vi "AVI Path Gen.vi"(8 "error in (no error)":errorcluster, 9 "Frames Per Second":u32=30, 11 "Output file path":path=path "C:/Users/Teo/Desktop/UCL Datasets/160915_13_48_57 FunctAcq-6 patches") -> (0 "error out":errorcluster, 2 "Codec used":string, 3 "AVI Refnum":T1)   [LabVIEW 2017]
uses:
  <vilib>/vision/Avi.llb/IMAQ AVI2 Refnum.ctl
  Globals/gl_8-bit montage window ctrl refs.vi
panel:
  out "name":string
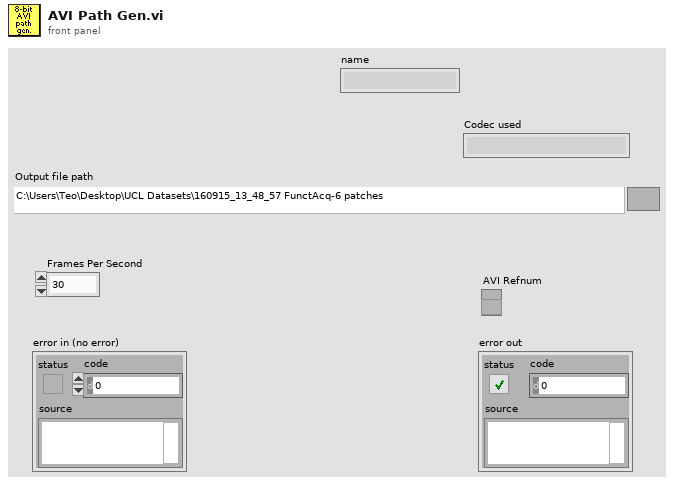
[diagram p1: front panel]
types:
  T1 = typedef "IMAQ AVI2 Refnum.ctl" = refnum<k20>
  T2 = typedef "8-bit video export window ctrl refs.ctl" = cluster{"This VI":refnum<vi>, "Add speed data":refnum<vi>, "Add camera videos":refnum<vi>, "Stop button":refnum<vi>, "Camera Video Adjustments":refnum<vi>, "Microscope Image Adjustments":refnum<vi>, "Execute":refnum<vi>, "Codec":refnum<vi>, "Channel to load":refnum<vi>, "Speed graph behaviour":refnum<vi>, "Include speed graph":refnum<vi>, "Number of rows to generate":refnum<vi>, "Path":refnum<vi>}
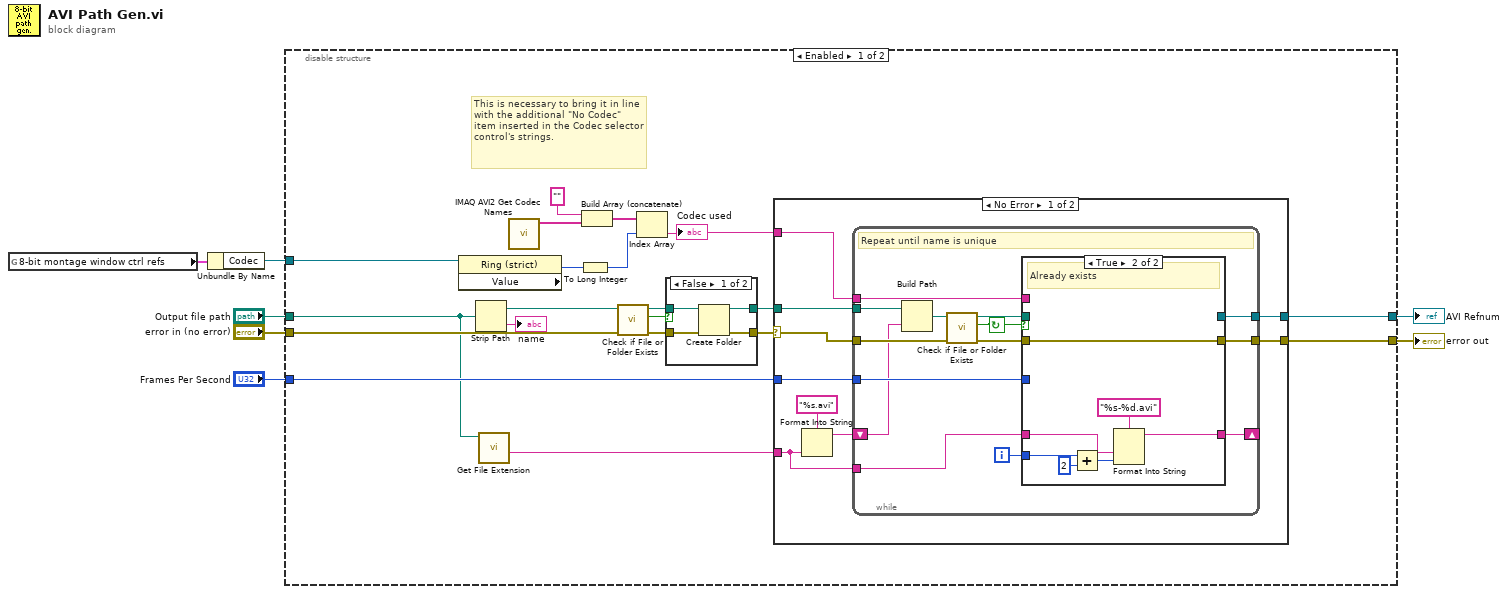
[diagram p0: block diagram]
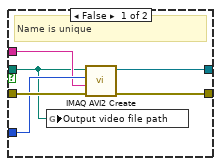
[diagram p2: hidden frame]
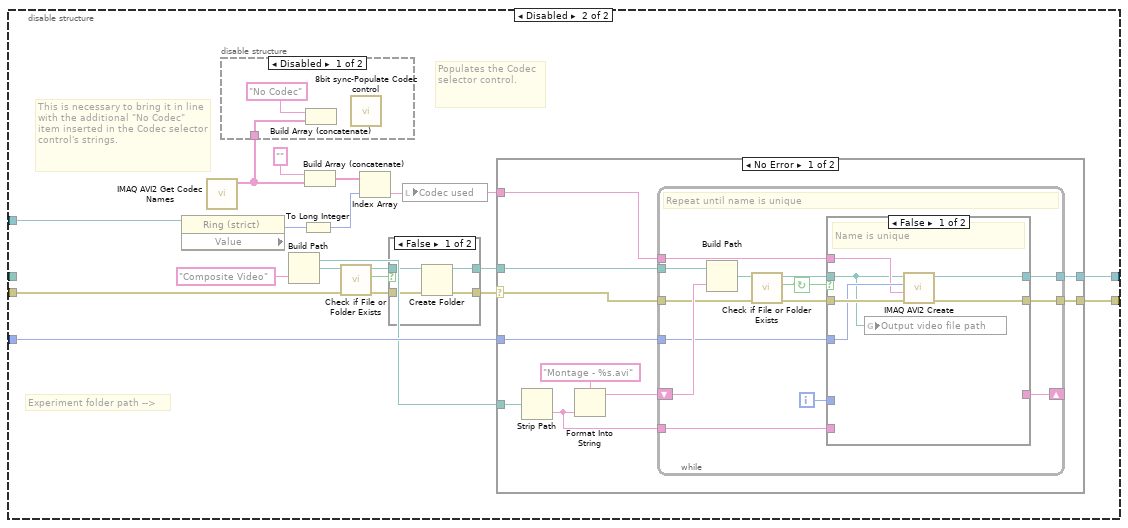
[diagram p5: hidden frame]
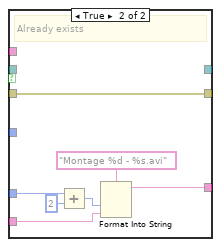
[diagram p7: hidden frame]
diagram:
  n1 = global read "gl_8-bit montage window ctrl refs.vi" "8-bit montage window ctrl refs"() -> (w3:T2)
  n2 = Unbundle By Name(w3) -> ("Codec"=w2:refnum<vi>)
  n3 = disable-structure shown="Enabled" {
    disable-tunnel: "Frames Per Second" -> [w22 w83]
    disable-tunnel: [w21 w82] -> w6
    disable-tunnel: "error in (no error)" -> [w19 w80]
    disable-tunnel: [w18 w79] -> w4
    disable-tunnel: w2 -> [w13 w75]
    disable-tunnel: "Output file path" -> [w9 _]
    frame Enabled {
      # "This is necessary to bring it in line with the additional \"No Codec\" item inserted in the Codec selector control's strings."
      n4 = property class="Ring (strict)"(reference=w13) -> ("Value"=w12:u16)  [unwired: 1 in, 2 out]
      n5 = Strip Path(path=w9) -> (stripped path=w27:path, name=→"name":string)
      n6 = call <vilib>:"Get File Extension.vi"("file"=w9) -> ("filename without extension"=w8:string)  [unwired: 6 in, 4 out]
      n7 = call "IMAQ AVI2 Get Codec Names"() -> ("Codec Names"=w15:string[])  [unwired: 10 in, 1 out]
      n8 = To Long Integer(number=w12) -> (32bit integer=w11:i32)
      n9 = Build Array (concatenate)("" ("Codec Name"), w15) -> (w14:string[])
      n10 = call <vilib>:"Check if File or Folder Exists.vi"("error in (no error)"=w19, "path"=w27) -> ("error out"=w26:errorcluster, "file or folder exists?"=w24:bool, "dup path"=w25:path)  [unwired: 7 in]
      n11 = Index Array(array=w14, index=w11) -> (element=w16:string)
      "Codec used" <- w16
      n12 = case shown="False" w24 {
        tunnel: w25 -> [w67 w70]
        tunnel: [w68 w70] -> w23
        tunnel: w26 -> [w66 w69]
        tunnel: [w65 w69] -> w20
        frame False {
          n13 = Create Folder(path (use dialog)=w67, error in=w66) -> (created path=w68:path, error out=w65:errorcluster)  [unwired: 1 in, 1 out]
        }
        frame True {
        }
      }
      n14 = case shown="No Error" w20 {
        selector: w20 -> [w30 w64]
        tunnel: w23 -> [w36 _]
        tunnel: w22 -> [w33 _]
        tunnel: [w32 _] -> w21
        tunnel: [w31 w64] -> w18
        tunnel: w16 -> [w29 _]
        tunnel: w8 -> [w28 _]
        frame No Error {
          n15 = Format Into String(format string="%s.avi", w28) -> (resulting string=w34:string)  [unwired: 2 in, 1 out]
          n16 = while {
            tunnel: w36 -> [w50]
            shift-right: [w42] -> _
            shift-left: w34 -> [w38]
            tunnel: w33 -> [w45]
            tunnel: [w44] -> w32
            tunnel: [w41] -> w31
            tunnel: w30 -> [w40]
            tunnel: w29 -> [w39]
            tunnel: w28 -> [w37]
            i -> [w43]
            stop <- w48 continue-if-true
            # "Repeat until name is unique"
            n17 = Build Path(base path=w50, name or relative path=w38) -> (appended path=w49:path)
            n18 = call <vilib>:"Check if File or Folder Exists.vi"("error in (no error)"=w40, "path"=w49) -> ("error out"=w46:errorcluster, "file or folder exists?"=w48:bool, "dup path"=w47:path)  [unwired: 7 in]
            n19 = case shown="True" w48 {
              tunnel: w47 -> [w51 _]
              tunnel: w46 -> [w56 w59]
              tunnel: w45 -> [w55 _]
              tunnel: [w54 _] -> w44
              tunnel: w43 -> [_ w61]
              tunnel: [_ w60] -> w42
              tunnel: [w53 w59] -> w41
              tunnel: w39 -> [w52 _]
              tunnel: w37 -> [_ w57]
              frame False {
                # "Name is unique"
                n20 = global write "gl_8-bit montage window ctrl refs.vi" "Output video file path"(w51) -> ()
                n21 = call "IMAQ AVI2 Create"("error in (no error)"=w56, "Codec"=w52, "Frames Per Second"=w55, "AVI Path"=w51) -> ("error out"=w53:errorcluster, "AVI Refnum"=w54:T1)  [unwired: 6 in]
              }
              frame True {
                # "Already exists"
                n22 = Add(x=w61, y=2) -> (x+y=w58:i32)
                n23 = Format Into String(format string="%s-%d.avi", w57, w58) -> (resulting string=w60:string)  [unwired: 2 in, 1 out]
              }
            }
          }
        }
        frame Error {
        }
      }
    }
    frame Disabled {
      # "Experiment folder path -->"
      # "Populates the Codec selector control."
      # "This is necessary to bring it in line with the additional \"No Codec\" item inserted in the Codec selector control's strings."
      n24 = property class="Ring (strict)"(reference=w75) -> ("Value"=w74:u16)  [unwired: 1 in, 2 out]
      n25 = call "IMAQ AVI2 Get Codec Names"() -> ("Codec Names"=w77:string[])  [unwired: 10 in, 1 out]
      n26 = disable-structure shown="Disabled" {
        disable-tunnel: w77 -> [w91 _]
        frame Disabled {
          n27 = Build Array (concatenate)("No Codec" ("Codec Name"), w91) -> ()  [unwired: 1 out]
          n28 = call "8bit sync-Populate Codec control.vi"() -> ()  [unwired: 11 in, 1 out]
        }
        frame Enabled {
        }
      }
      n29 = To Long Integer(number=w74) -> (32bit integer=w73:i32)
      n30 = Build Array (concatenate)("" ("Codec Name"), w77) -> (w76:string[])
      n31 = Index Array(array=w76, index=w73) -> (element=w72:string)
      n32 = local write "Codec used"(w72) -> ()
      n33 = Build Path(base path=w71, name or relative path="Composite Video") -> (appended path=w89:path)
      n34 = call <vilib>:"Check if File or Folder Exists.vi"("error in (no error)"=w80, "path"=w89) -> ("error out"=w88:errorcluster, "file or folder exists?"=w86:bool, "dup path"=w87:path)  [unwired: 7 in]
      n35 = case shown="False" w86 {
        tunnel: w87 -> [w132 w135]
        tunnel: [w133 w135] -> w84
        tunnel: w88 -> [w131 w134]
        tunnel: [w130 w134] -> w81
        frame False {
          n36 = Create Folder(path (use dialog)=w132, error in=w131) -> (created path=w133:path, error out=w130:errorcluster)  [unwired: 1 in, 1 out]
        }
        frame True {
        }
      }
      n37 = case shown="No Error" w81 {
        selector: w81 -> [w93 w129]
        tunnel: w84 -> [w101 _]
        tunnel: [w100 _] -> w71
        tunnel: w83 -> [w97 _]
        tunnel: [w95 _] -> w82
        tunnel: [w94 w129] -> w79
        tunnel: w72 -> [w92 _]
        frame No Error {
          n38 = Strip Path(path=w100) -> (name=w96:string)  [unwired: 1 out]
          n39 = Format Into String(format string="Montage - %s.avi", w96) -> (resulting string=w98:string)  [unwired: 2 in, 1 out]
          n40 = while {
            tunnel: w101 -> [w115]
            shift-right: [w105] -> _
            shift-left: w98 -> [w114]
            tunnel: w97 -> [w109]
            tunnel: [w108] -> w95
            tunnel: w96 -> [w107]
            tunnel: [w104] -> w94
            tunnel: w93 -> [w103]
            tunnel: w92 -> [w102]
            i -> [w106]
            stop <- w112 continue-if-true
            # "Repeat until name is unique"
            n41 = Build Path(base path=w115, name or relative path=w114) -> (appended path=w113:path)
            n42 = call <vilib>:"Check if File or Folder Exists.vi"("error in (no error)"=w103, "path"=w113) -> ("error out"=w110:errorcluster, "file or folder exists?"=w112:bool, "dup path"=w111:path)  [unwired: 7 in]
            n43 = case shown="False" w112 {
              tunnel: w111 -> [w116 _]
              tunnel: w110 -> [w121 w122]
              tunnel: w109 -> [w120 _]
              tunnel: [w119 _] -> w108
              tunnel: w107 -> [_ w124]
              tunnel: w106 -> [_ w125]
              tunnel: [_ w123] -> w105
              tunnel: [w118 w122] -> w104
              tunnel: w102 -> [w117 _]
              frame False {
                # "Name is unique"
                n44 = global write "gl_8-bit montage window ctrl refs.vi" "Output video file path"(w116) -> ()
                n45 = call "IMAQ AVI2 Create"("error in (no error)"=w121, "Codec"=w117, "Frames Per Second"=w120, "AVI Path"=w116) -> ("error out"=w118:errorcluster, "AVI Refnum"=w119:T1)  [unwired: 6 in]
              }
              frame True {
                # "Already exists"
                n46 = Add(x=w125, y=2) -> (x+y=w126:i32)
                n47 = Format Into String(format string="Montage %d - %s.avi", w126, w124) -> (resulting string=w123:string)  [unwired: 2 in, 1 out]
              }
            }
          }
        }
        frame Error {
        }
      }
    }
  }
  "AVI Refnum" <- w6
  "error out" <- w4
